vi "PanelWizard_FindButtonRef.vi"(8 "error in (no error)":errorcluster, 10 "ButtonRefs":refnum<vi>[](array[refnum]), 11 "Display State In":T1={"DisplayStyle"=enum."3D Style", "LaunchType"=enum."LaunchHDV", "UserVIPath"=path "", "Button Text"="", "UseDefaultButtonText?"=TRUE, "Run User VI?"=TRUE, "CommandLine"="", "StandardInput"="", "Working Directory"=path ""} caption="State") -> (0 "error out":errorcluster, 1 "Disabled Buttons [ref]":refnum<vi>[](array[refnum]), 2 "Enabled Button (ref)":refnum<vi>, 3 "Display State Out":T1={"DisplayStyle"=enum."3D Style", "LaunchType"=enum."LaunchHDV", "UserVIPath"=path "", "Button Text"="", "UseDefaultButtonText?"=TRUE, "Run User VI?"=TRUE, "CommandLine"="", "StandardInput"="", "Working Directory"=path ""} caption="State")   [LabVIEW 2012, in "PanelWizard.xctl"]
uses:
  PanelWizard.xctl
  PanelWizard_State.ctl
  PanelWizard_DisplayType.ctl
  PanelWizard_LaunchOptions.ctl
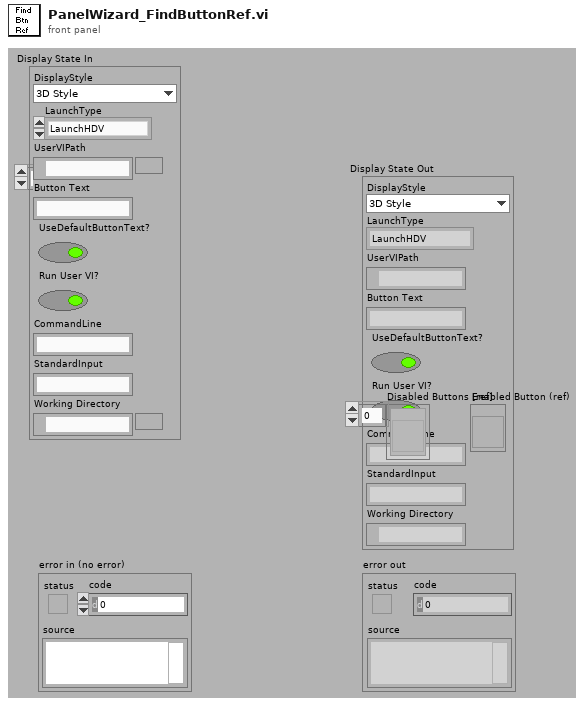
[diagram p1: front panel]
types:
  T1 = typedef "PanelWizard.xctl/PanelWizard_State.ctl" = cluster{"DisplayStyle":T2, "LaunchType":T3, "UserVIPath":path, "Button Text":string, "UseDefaultButtonText?":bool, "Run User VI?":bool, "CommandLine":string, "StandardInput":string, "Working Directory":path}
  T2 = typedef "PanelWizard.xctl/PanelWizard_DisplayType.ctl" = enum16{"3D Style", "LabVIEW Classic Style", "System Style"}
  T3 = typedef "PanelWizard.xctl/PanelWizard_LaunchOptions.ctl" = enum16{"LaunchHDV", "LaunchSVMonitor", "LaunchUserVI", "Run command line"}
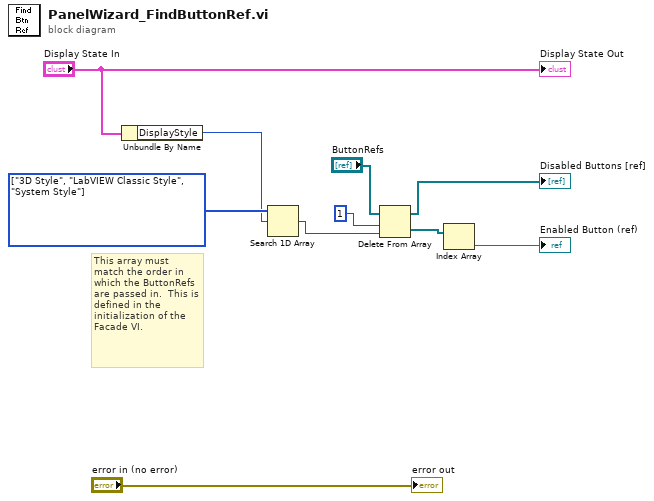
[diagram p0: block diagram]
diagram:
  w8 = T2[] [enum."3D Style", enum."LabVIEW Classic Style", enum."System Style"] items=["3D Style", "LabVIEW Classic Style", "System Style"]
  # "This array must match the order in which the ButtonRefs are passed in.  This is defined in the initialization of the Facade VI."
  n1 = Unbundle By Name("Display State In") -> ("DisplayStyle"=w7:T2)
  n2 = Search 1D Array(1D array=w8, element=w7) -> (index of element=w5:i32)  [unwired: 1 in]
  n3 = Delete From Array(array="ButtonRefs", length=1, index=w5) -> (deleted portion=w2:refnum<vi>[], array with subset deleted=→"Disabled Buttons [ref]":refnum<vi>[])
  n4 = Index Array(array=w2) -> (element=→"Enabled Button (ref)":refnum<vi>)  [unwired: 1 in]
  "Display State Out" <- "Display State In"
  "error out" <- "error in (no error)"
